vi "Test.vi"() -> ()   [LabVIEW 2019, in "LabSSH.lvlib"]
doc: "<License>This software is distributed under the BSD 3-Clause License. For the full license please see license.txt or visit www.labvolution.com/license</License>"
uses:
  LabSSH.lvlib
  Connection Info..cluster.ctl
  Password..cluster.ctl
  Private Public Key..cluster.ctl
  connect_password.vi
  connect_key.vi
panel:
  in  "Connection Info.":T1={"IP地址"="192.168.1.106", "用户名"="pi", "端口 (22)"=22}
  in  "Password":T2={"密码"="zjl"}
  in  "Connection Type":enum16{"Password", "Private Key"}(ring)
  in  "Private_Public Key":T3
  in  "Expected Response":string="raspberrypi："
  out "isSshConnected":bool
  out "SSH Response":string="SSH connection closed\r\n"
  in  "采集时间":i32=10
  in  "采集命令":string="cd /home/pi/leakad\nls\nsudo ./ADS1256 0 2000 5 1"
  in  "关闭":bool
  in  "连接设备":bool
  in  "error in (no error)":errorcluster
  out "Output":string="Linux raspberrypi 4.19.97-v7+ #1294 SMP Thu Jan 30 13:15:58 GMT 2020 armv7l\r\n\r\nThe programs included with the Debian GNU/Linux system are free software;\r\nthe exact distribution terms for each program are described in the\r\nindividual files in /usr/share/doc/*/copyright.\r\n\r\nDebian GNU/Linux comes with ABSOLUTELY NO WARRANTY, to the extent\r\npermitted by applicable law.\r\nLast login: Sun Apr 26 10:17:10 2020\r\r\npi@raspberrypi:~$ cd /home/pi/leakad\r\npi@raspberrypi:~/leakad$ ls\r\nADS1256  datafile.dat\r\npi@raspberrypi:~/leakad$ sudo ./ADS1256 0 2000 5 1\r\npi@raspberrypi:~/leakad$ "
  # "C:\\\\Working Folder\\\\ssh.git\\\\LabSSH\\\\raspberrypi_private_openssh.ppk"
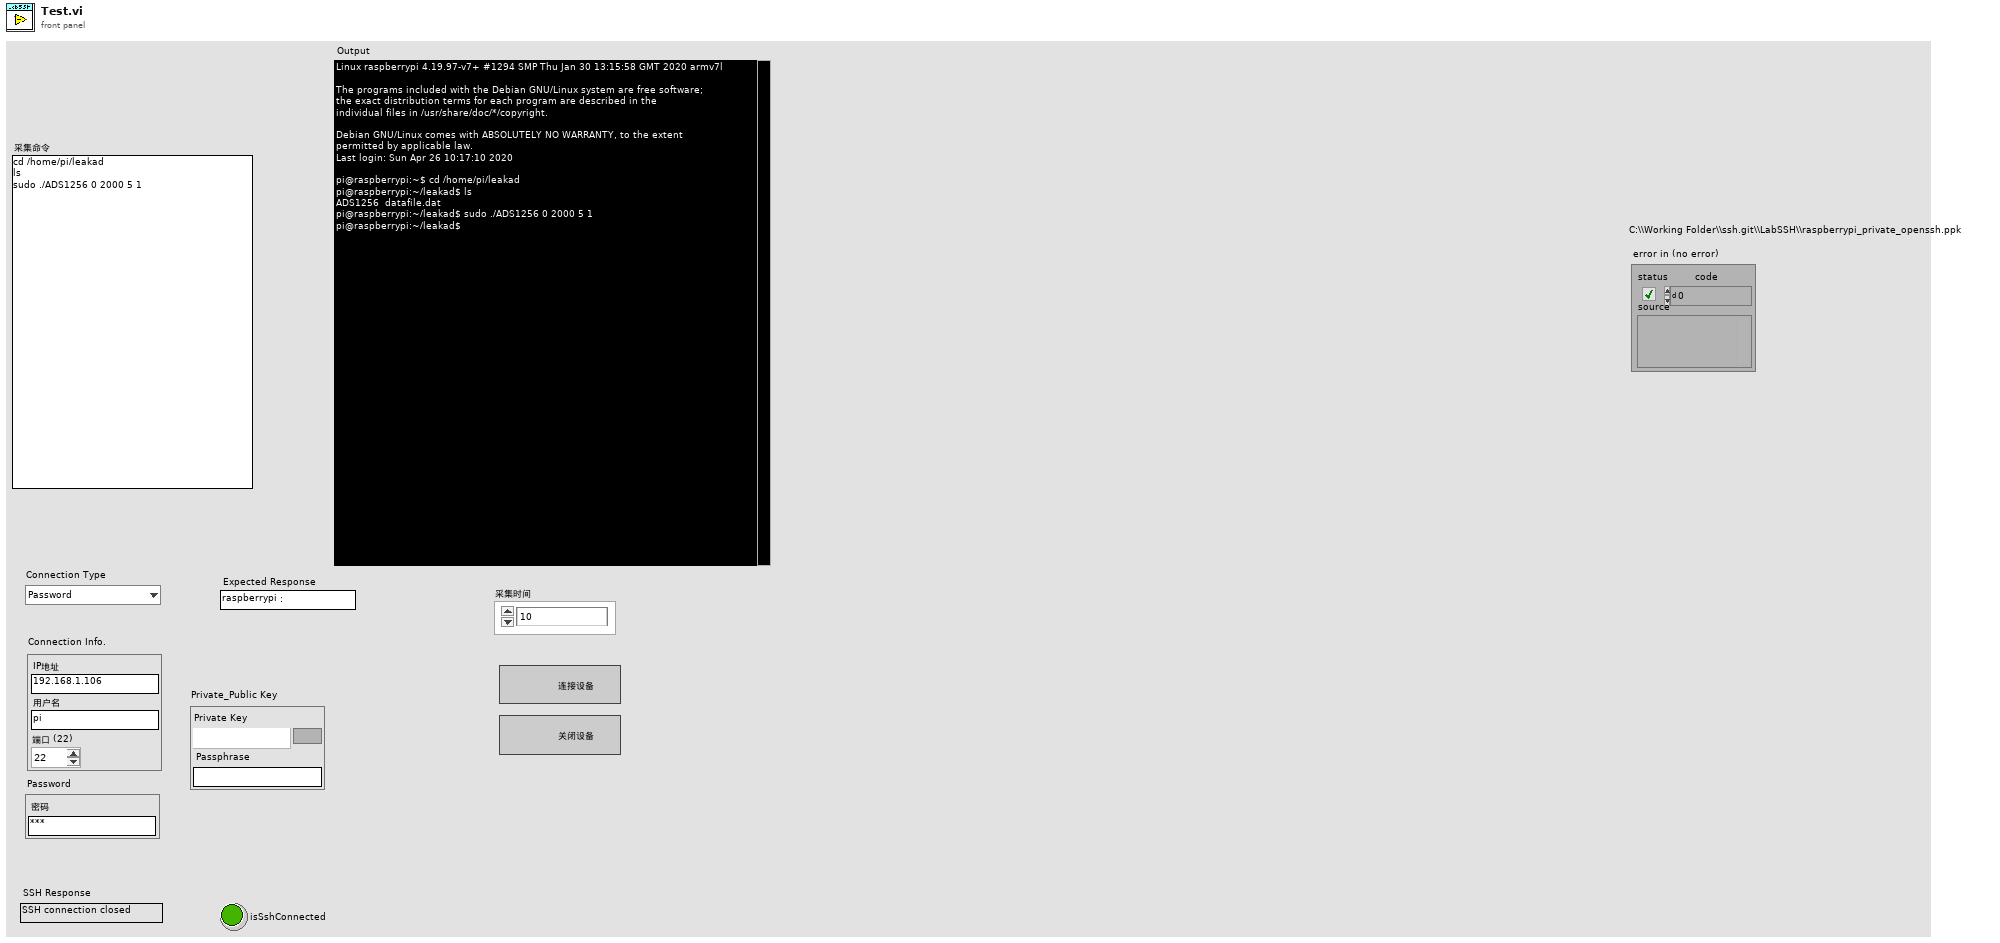
[diagram p1: front panel]
types:
  T1 = typedef "LabSSH.lvlib/Connection Info..cluster.ctl" = cluster{"IP地址":string, "用户名":string, "端口 (22)":i32}
  T2 = typedef "LabSSH.lvlib/Password..cluster.ctl" = cluster{"密码":string}
  T3 = typedef "LabSSH.lvlib/Private Public Key..cluster.ctl" = cluster{"Private Key":path, "Passphrase":string}
  T4 = enum32{"invalid app kind", "Development System", "Run Time System", "Student Edition", "Embedded LabVIEW", "Evaluation", "Custom"}
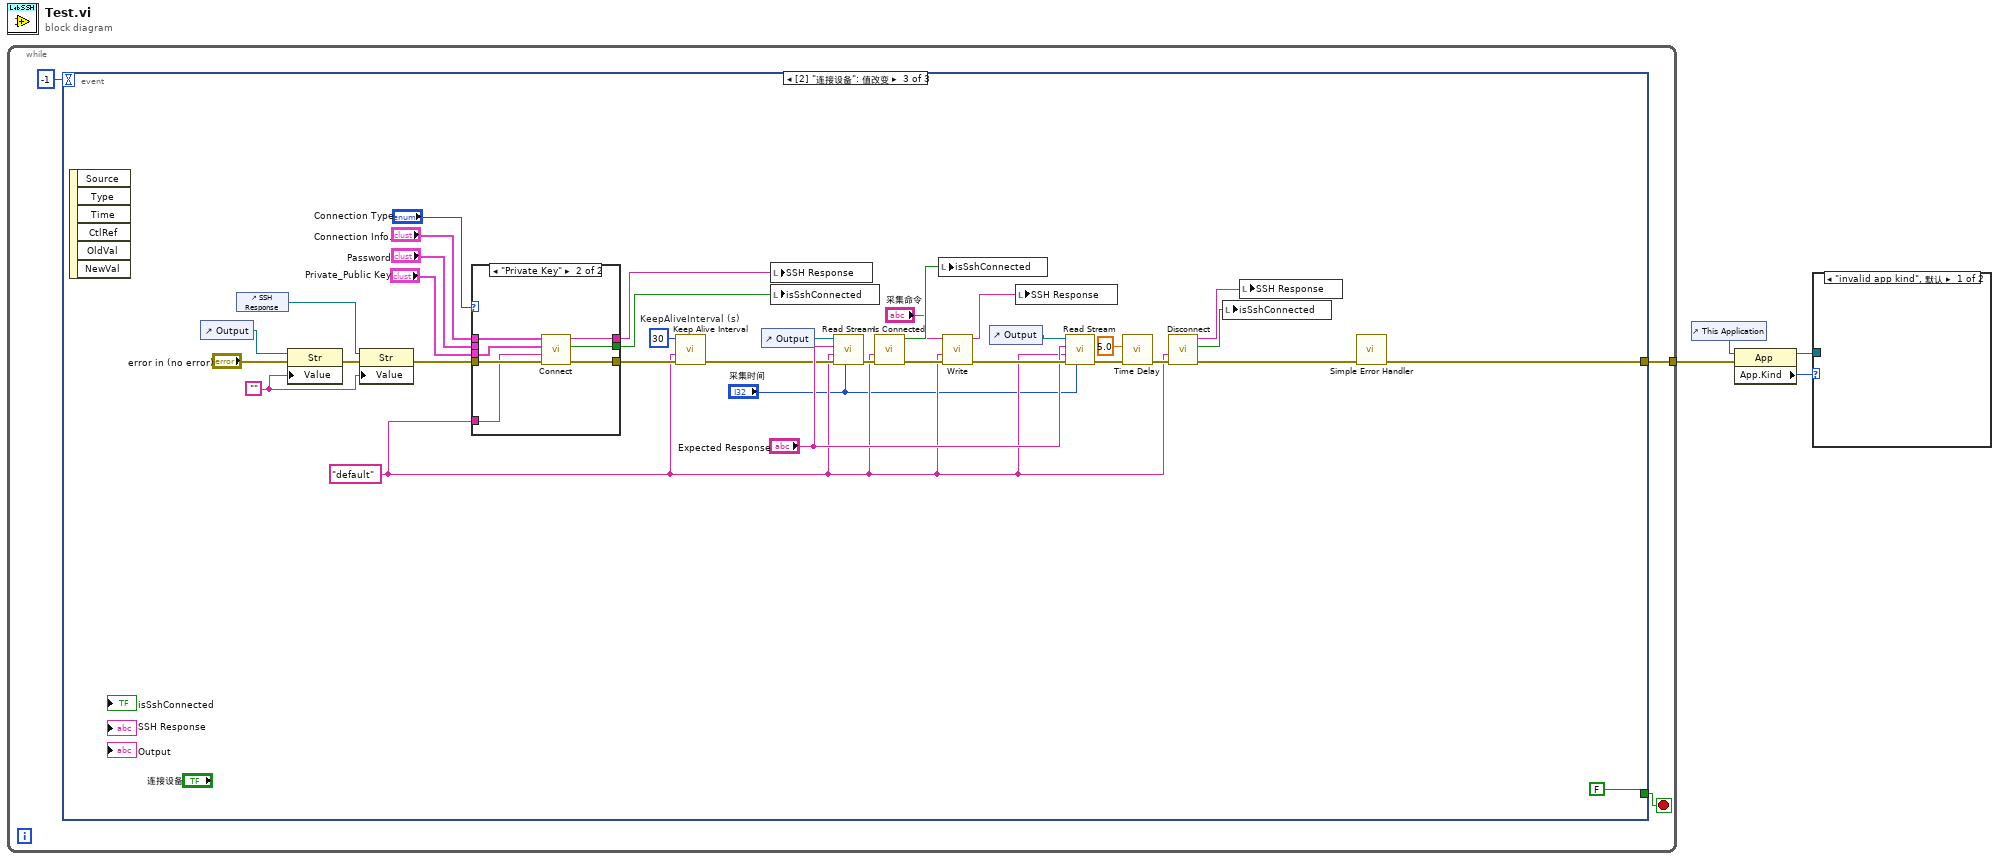
[diagram p0: block diagram]
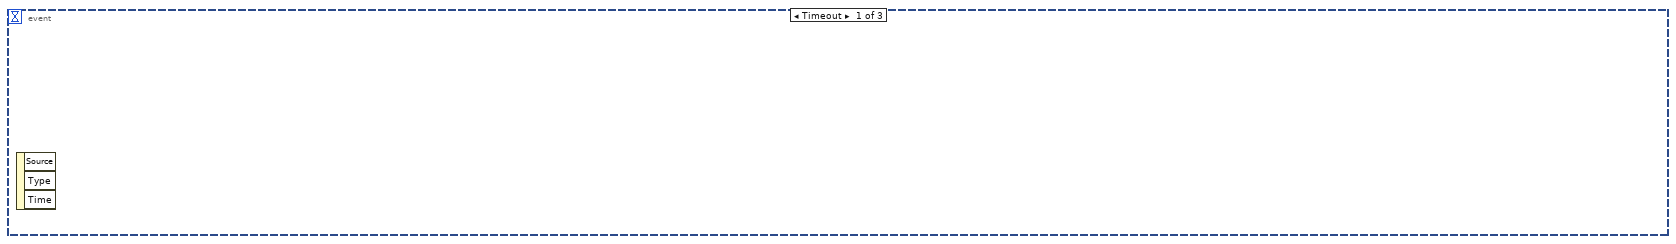
[diagram p2: hidden frame]
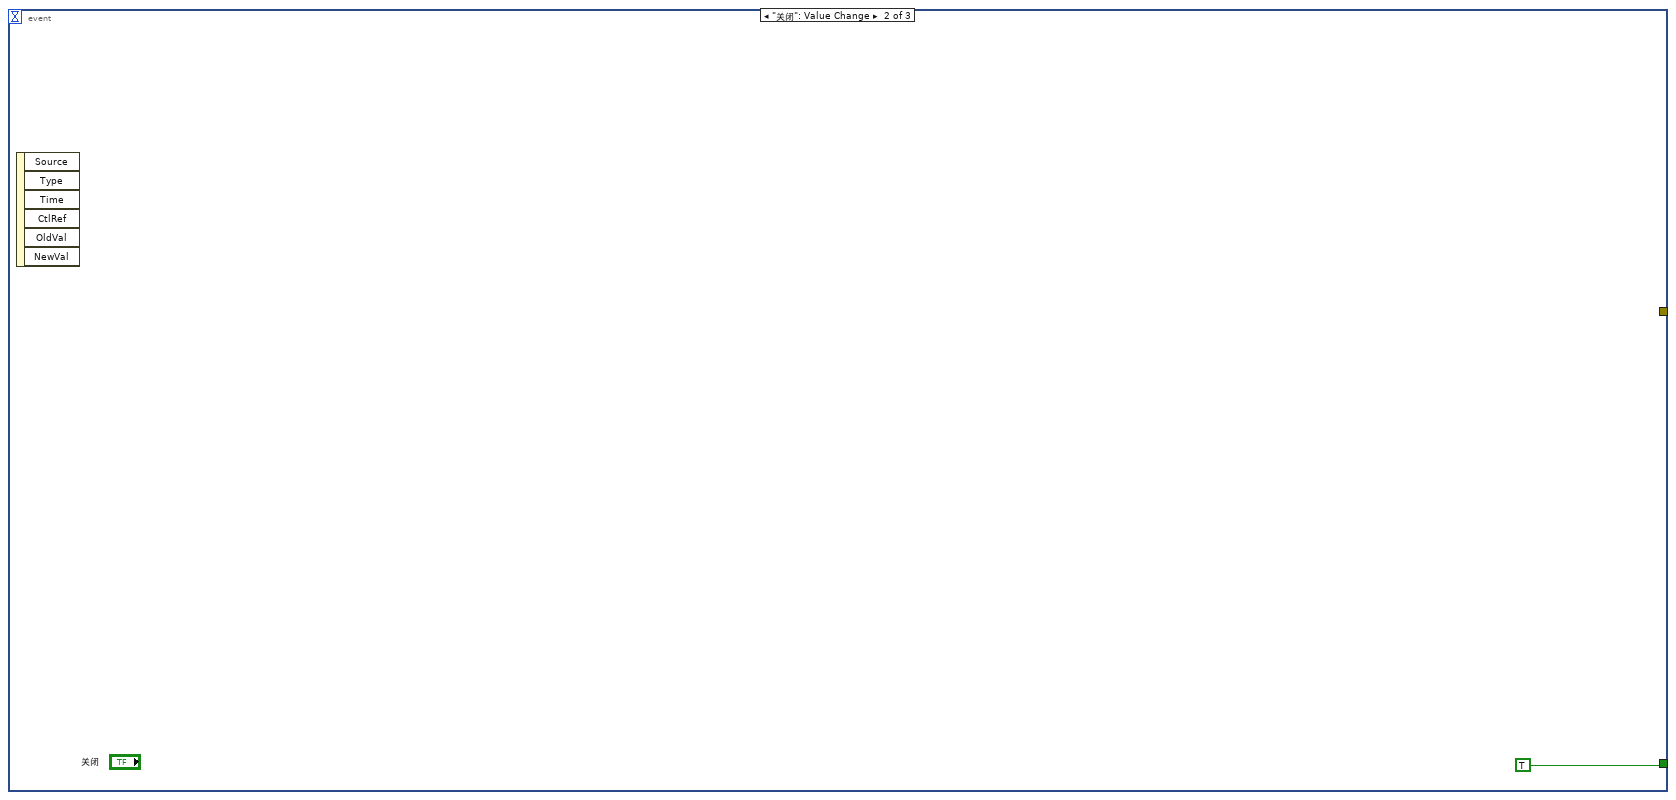
[diagram p3: hidden frame]
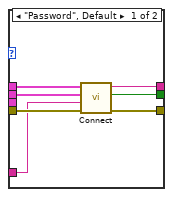
[diagram p4: hidden frame]
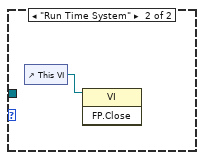
[diagram p5: hidden frame]
diagram:
  n1 = while {
    tunnel: [w6] -> w3
    stop <- w7 stop-if-true
    n2 = event shown="[2] \"连接设备\": 值改变" {
      selector: _ -> [_ _ _]
      dyn-events: _ -> [_ _ _]
      timeout: -1 -> [_ _ _]
      tunnel: [_ TRUE FALSE] -> w7
      tunnel: [_ _ w17] -> w6
      event Timeout {
        n3 = event-data() -> ()  [unwired: 1 in, 3 out]
      }
      event "关闭": Value Change {
        n4 = event-data() -> ()  [unwired: 1 in, 6 out]
      }
      event "连接设备": Value Change {
        w10 = "default" ("Connection Name")
        w14 = 30  # KeepAliveInterval (s)
        w25 = ""
        n5 = event-data() -> ()  [unwired: 1 in, 6 out]
        n6 = control-ref of="Output"() -> (w28:refnum<vi>)
        n7 = control-ref of="SSH Response"() -> (w26:refnum<vi>)
        n8 = property class="Str"(reference=w28, error in="error in (no error)", "Value"=w25) -> (error out=w29:errorcluster)  [unwired: 1 out]
        n9 = property class="Str"(reference=w26, error in=w29, "Value"=w25) -> (error out=w27:errorcluster)  [unwired: 1 out]
        n10 = case shown="\"Private Key\"" "Connection Type" {
          tunnel: [w49 w54] -> w15
          tunnel: "Connection Info." -> [w48 w56]
          tunnel: "Password" -> [w47 _]
          tunnel: [w46 w53] -> w37
          tunnel: [w45 w52] -> w32
          tunnel: w27 -> [w44 w55]
          tunnel: "Private_Public Key" -> [_ w51]
          tunnel: w10 -> [w43 w50]
          frame "Password", Default {
            n11 = call-poly "Connect.vi"("error in (no error)"=w44, "Connection Name"=w43, "Password"=w47, "Connection Info."=w48) -> ("error out"=w49:errorcluster, "isSshConnected"=w46:bool, "Return String"=w45:string)  [unwired: 5 in]
          }
          frame "Private Key" {
            n12 = call-poly "Connect.vi"("error in (no error)"=w55, "Connection Name"=w50, "Private_Public Key"=w51, "Connection Info."=w56) -> ("error out"=w54:errorcluster, "isSshConnected"=w53:bool, "Return String"=w52:string)  [unwired: 5 in]
          }
        }
        n13 = call "Keep Alive Interval.vi"("error in (no error)"=w15, "Connection Name"=w10, "KeepAliveInterval (s)"=w14) -> ("error out"=w16:errorcluster)  [unwired: 8 in]
        n14 = control-ref of="Output"() -> (w42:refnum<vi>)
        n15 = local write "SSH Response"(w32) -> ()
        n16 = local write "isSshConnected"(w37) -> ()
        n17 = call "Read Stream.vi"("Timout (s)"="采集时间", "error in (no error)"=w16, "Connection Name"=w10, "Expected Response"="Expected Response", "Output ref"=w42) -> ("error out"=w38:errorcluster)  [unwired: 6 in]
        n18 = call "Is Connected.vi"("error in (no error)"=w38, "Connection Name"=w10) -> ("error out"=w35:errorcluster, "isSshConnected"=w36:bool)  [unwired: 8 in]
        n19 = local write "isSshConnected"(w36) -> ()
        n20 = call "Write.vi"("error in (no error)"=w35, "Connection Name"=w10, "Command"="采集命令") -> ("error out"=w33:errorcluster, "Return String"=w31:string)  [unwired: 7 in]
        n21 = control-ref of="Output"() -> (w34:refnum<vi>)
        n22 = local write "SSH Response"(w31) -> ()
        n23 = call "Read Stream.vi"("Timout (s)"="采集时间", "error in (no error)"=w33, "Connection Name"=w10, "Expected Response"="Expected Response", "Output ref"=w34) -> ("error out"=w20:errorcluster)  [unwired: 6 in]
        n24 = call "Time Delay"("error in (no error)"=w20, "Delay Time (s)"=5.0) -> ("error out"=w19:errorcluster)  [unwired: 9 in]
        n25 = call "Disconnect.vi"("error in (no error)"=w19, "Connection Name"=w10) -> ("error out"=w30:errorcluster, "isSshConnected"=w12:bool, "Return String"=w13:string)  [unwired: 7 in]
        n26 = local write "isSshConnected"(w12) -> ()
        n27 = local write "SSH Response"(w13) -> ()
        n28 = call <vilib>:"Simple Error Handler.vi"("error in (no error)"=w30) -> ("error out"=w17:errorcluster)  [unwired: 4 in, 4 out]
      }
    }
  }
  n29 = control-ref of="This Application"() -> (w4:refnum<vi>)
  n30 = property class="App"(reference=w4, error in=w3) -> (reference out=w1:refnum<vi>, "App.Kind"=w2:T4)  [unwired: 1 out]
  n31 = case shown="\"invalid app kind\", 默认" w2 {
    tunnel: w1 -> [_ _]
    frame "invalid app kind", Default {
    }
    frame "Run Time System" {
      n32 = control-ref of="This VI"() -> (w57:refnum<vi>)
      n33 = invoke class="VI" method="FP.Close"(reference=w57) -> ()  [unwired: 2 in, 3 out]
    }
  }
